vi "read_string.vi"(8 "error in (no error)":errorcluster, 11 "VISA resource name 2":refnum<visa-resource-name>) -> (0 "error out":errorcluster, 2 "read buffer":string, 3 "VISA resource name":refnum<visa-resource-name>)   [LabVIEW 2021]
panel:
  out "error?":bool
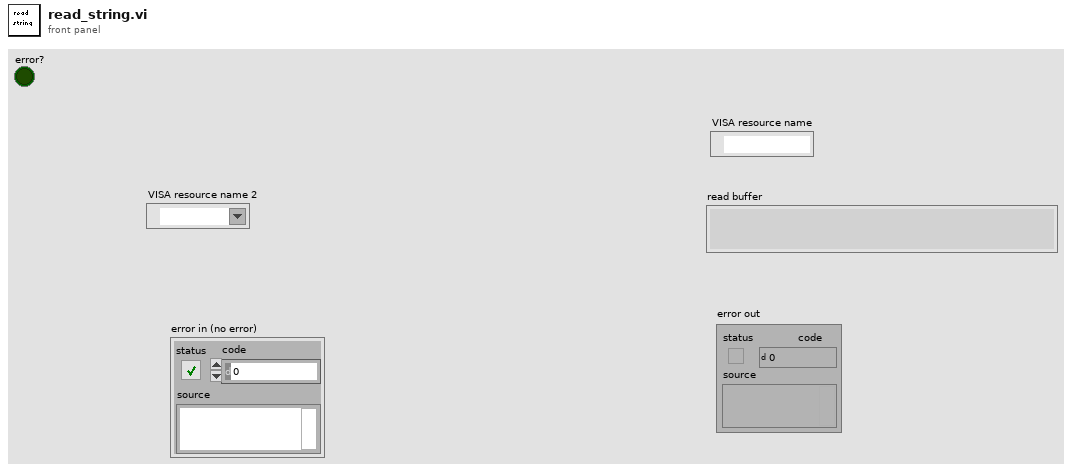
[diagram p1: front panel]
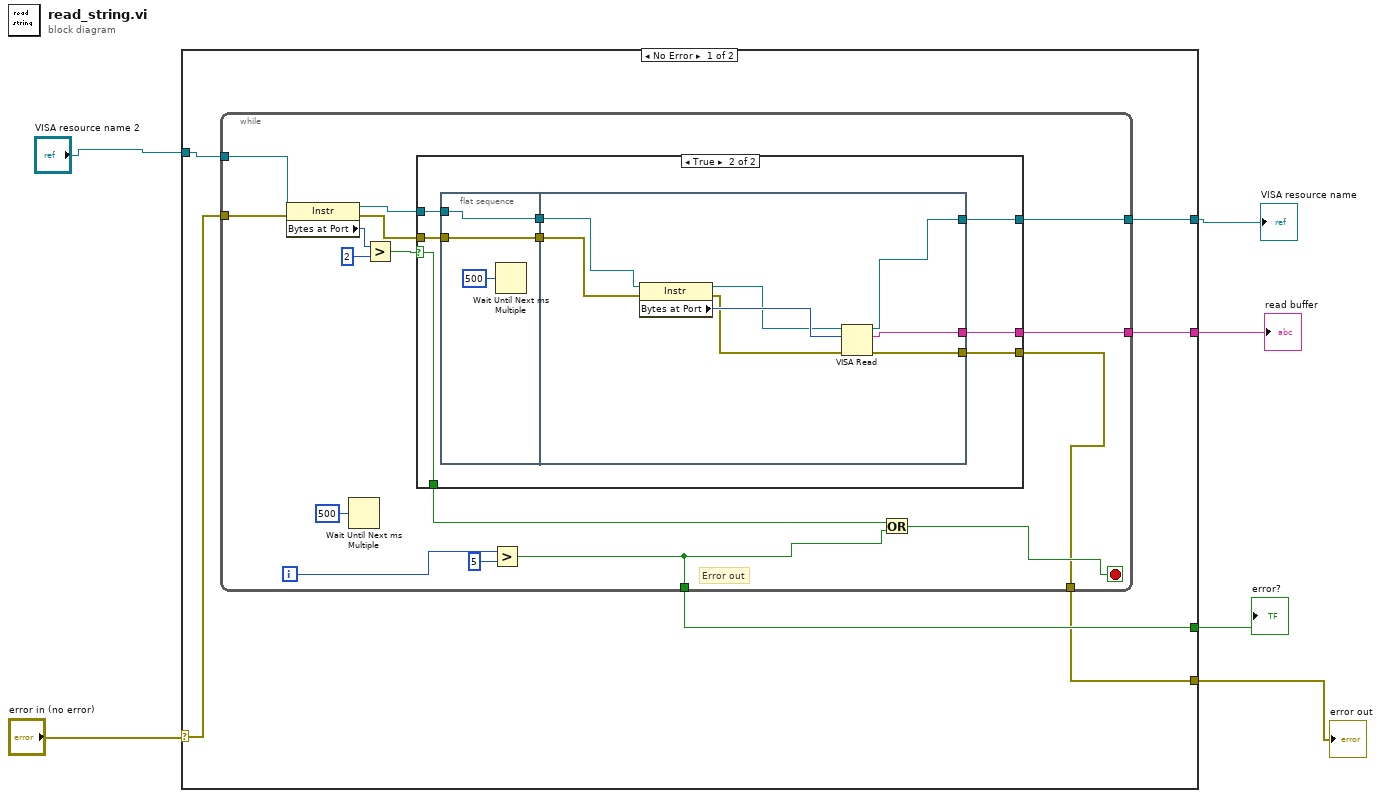
[diagram p0: block diagram]
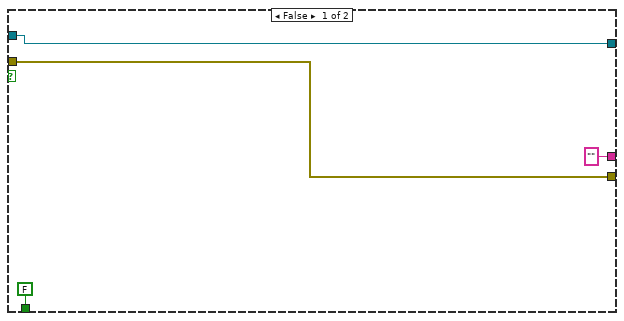
[diagram p2: hidden frame]
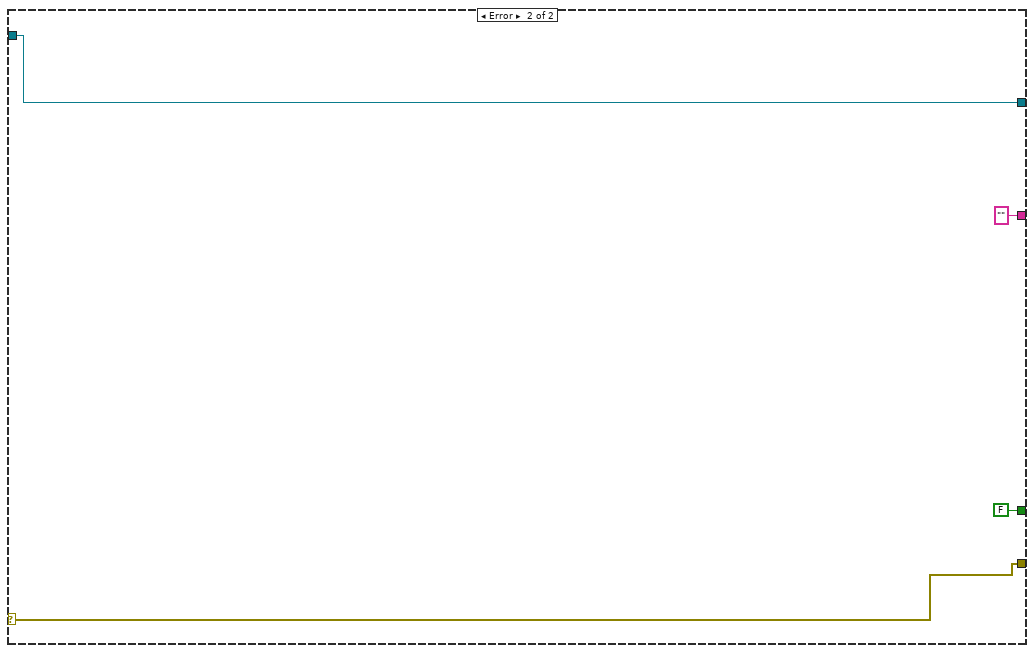
[diagram p3: hidden frame]
diagram:
  n1 = case shown="No Error" "error in (no error)" {
    selector: "error in (no error)" -> [w8 w55]
    tunnel: "VISA resource name 2" -> [w12 w52]
    tunnel: [w11 "" ("read buffer")] -> w6
    tunnel: [w10 FALSE] -> w5
    tunnel: [w9 w52] -> w4
    tunnel: [w7 w55] -> w2
    frame No Error {
      n2 = while {
        tunnel: w12 -> [w23]
        tunnel: [w18] -> w10
        tunnel: [w17] -> w11
        tunnel: [w16] -> w9
        tunnel: w8 -> [w15]
        tunnel: [w13] -> w7
        i -> [w21]
        stop <- w19 stop-if-true
        # "Error out"
        n3 = property class="Instr"(reference=w23, error in=w15) -> (reference out=w24:refnum<visa-resource-name>, error out=w14:errorcluster, "Bytes at Port"=w26:u32)
        n4 = Wait Until Next ms Multiple(millisecond multiple=u32 500) -> ()  [unwired: 1 out]
        n5 = Greater?(x=w26, y=u32 2) -> (0:w25:bool)
        n6 = case shown="True" w25 {
          selector: w25 -> [_ w38]
          tunnel: w24 -> [w30 w39]
          tunnel: [FALSE w38] -> w22
          tunnel: ["" ("read buffer") w37] -> w17
          tunnel: [w30 w36] -> w16
          tunnel: w14 -> [w29 w34]
          tunnel: [w29 w33] -> w13
          frame False {
          }
          frame True {
            n7 = flat-sequence {
              tunnel: [w42] -> w40
              tunnel: w39 -> [w42]
              tunnel: [w41] -> w35
              tunnel: w34 -> [w41]
              tunnel: w40 -> [w51]
              tunnel: [w48] -> w37
              tunnel: [w47] -> w36
              tunnel: w35 -> [w46]
              tunnel: [w44] -> w33
              frame #0 {
                n8 = Wait Until Next ms Multiple(millisecond multiple=u32 500) -> ()  [unwired: 1 out]
              }
              frame #1 {
                n9 = property class="Instr"(reference=w51, error in=w46) -> (reference out=w49:refnum<visa-resource-name>, error out=w45:errorcluster, "Bytes at Port"=w50:u32)
                n10 = VISA Read(VISA resource name=w49, byte count=w50, error in (no error)=w45) -> (VISA resource name out=w47:refnum<visa-resource-name>, read buffer=w48:string, error out=w44:errorcluster)  [unwired: 1 out]
              }
            }
          }
        }
        n11 = Greater?(x=w21, y=5) -> (0:w18:bool)
        n12 = Or(x=w22, y=w18) -> (x .or. y?=w19:bool)
      }
    }
    frame Error {
    }
  }
  "read buffer" <- w6
  "error?" <- w5
  "VISA resource name" <- w4
  "error out" <- w2
